vi "AB_API Can Add.vi"(7 "top tree? (true)":bool=TRUE, 8 "error in (no error)":errorcluster, 10 "AB_Source in":refnum<class "AB_Source.lvclass">, 11 "Build in":refnum<class "AB_Build.lvclass">) -> (0 "error out":errorcluster, 1 "can add?":bool, 2 "AB_Source out":refnum<class "AB_Source.lvclass">, 3 "Build out":refnum<class "AB_Build.lvclass">)   [LabVIEW 2020]
uses:
  <vilib>/AppBuilder/AB_Classes/Source/AB_Source.lvclass
  <vilib>/AppBuilder/AB_Classes/Build/AB_Build.lvclass
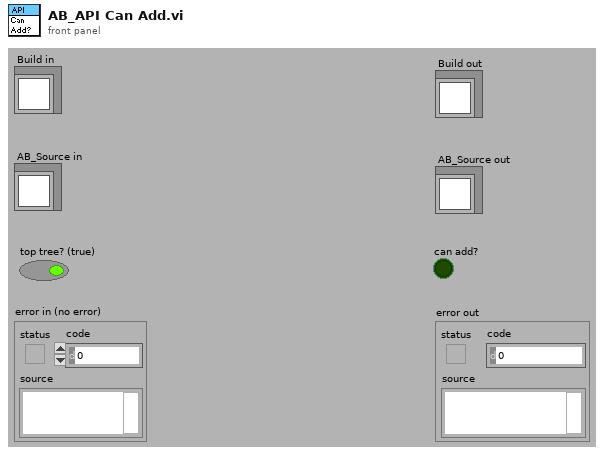
[diagram p1: front panel]
types:
  T1 = typedef "AB_Source.ctl" = cluster{"path":path, "itemID":string, "parentIndex":i32, "sourceInclusion":T2, "destinationIndex":i32, "properties":T3[], "newName":string, "lvfile":bool, "valid":bool, "eng_inBuild":bool, "eng_isNonVILink":bool, "Amalgamation":bool, "Amalgamation Piece":bool, "eng_delimitedName":string, "preventRename":bool}
  T2 = typedef "AB_Source_Inclusion.ctl" = enum16{"IncludeIfReferenced", "Include", "Exclude", "TopLevel"}
  T3 = typedef "AB_Source_Properties.ctl" = cluster{"sourcePropertyType":T4, "value":variant}
  T4 = typedef "AB_Source_Property_Type.ctl" = enum16{"Remove block diagram", "Remove front panel", "Password", "Window has title bar", "Show menu bar", "Show vertical scroll bar", "Show horizontal scroll bar", "Show toolbar", "Show Abort button", "Show fp when called", "Window behavior", "Allow user to close window", "Window run-time position", "Run when opened", "Allow debugging", "Auto error handling", "Generate guard code", "Use stack variables", "Expression folding", "Integer only", "Inline subVI"}
  T5 = typedef "AB_Build.ctl" = cluster{"buildSpecName":string, "buildSpecDescription":string, "destinations":refnum<class "AB_Destination.lvclass">[], "exclusionOption":T6, "defaultLanguage":string, "supportedLanguages":string[], "excludedDirectories":path[], "buildContext":refnum<vi>, "buildObject":T7, "preview":bool, "programatic":bool, "progressBarEvents":T8, "userLog_Path":path, "preActionID":string, "preAction_Path":path, "postActionID":string, "postAction_Path":path, "eng_checkForBrokenVIs?":bool, "eng_verboseLinkerErrors?":bool, "localDest_Path":path, "targetDest_Path":path, "removeVIObject":u16, "cache":refnum<class "PreviewCache.lvclass">, "use cache":bool, "previewCache_ID":string, "buildCache_ID":string, "eng_TempLocalDest_Path":path, "eng_collectDependencies?":bool, "versionInfo":cluster{"buildVersion":cluster{"major":u16, "minor":u16, "patch":u16, "build":u16}, "autoIncrement":bool}, "eng_enableVIChecksums":bool}
  T6 = typedef "AB_Exclusion_Option.ctl" = cluster{"typedefs":bool, "polymorphicVIs":bool, "unusedLibraryItems":bool, "modifyLibraryFile":bool, "edit-timeDependencies":bool, "inlineVIs":bool, "dependent PPLs":bool, "dependent DLLs":bool}
  T7 = typedef "ItemRef.ctl" = u64
  T8 = typedef "provcom_ProgressBar_Events.ctl" = cluster{"newJob":refnum<user-event>, "newItem":refnum<user-event>, "errorMsg":T9, "cancel":refnum<user-event>}
  T9 = typedef "mxLvBuildError.ctl" = refnum<user-event>
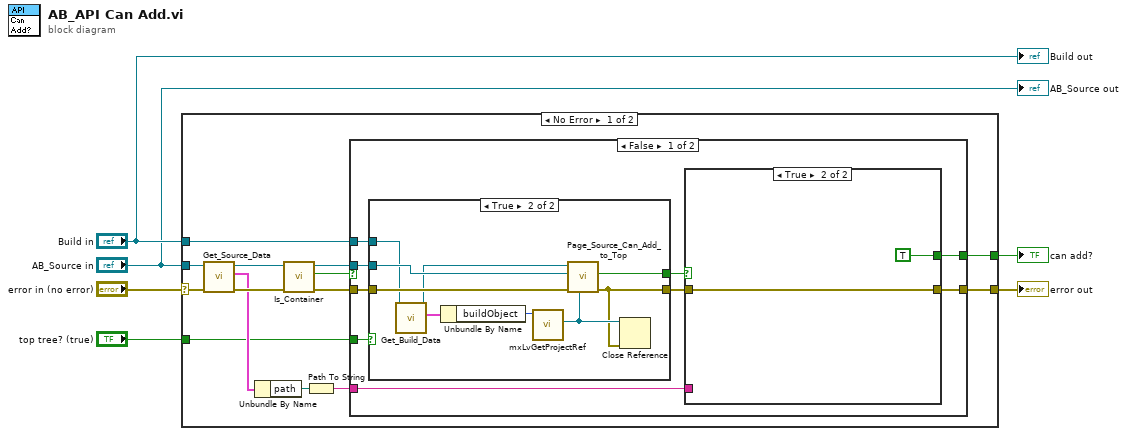
[diagram p0: block diagram]
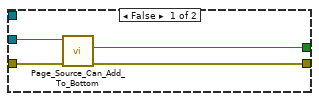
[diagram p2: hidden frame]
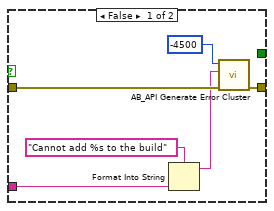
[diagram p3: hidden frame]
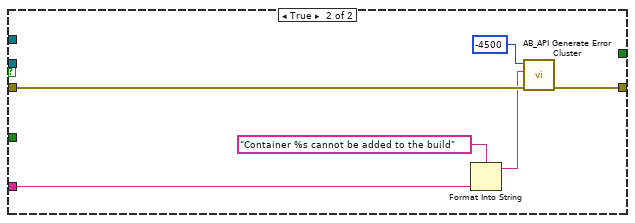
[diagram p4: hidden frame]
diagram:
  n1 = case shown="No Error" "error in (no error)" {
    selector: "error in (no error)" -> [w13 w57]
    tunnel: "Build in" -> [w17 _]
    tunnel: "AB_Source in" -> [w16 _]
    tunnel: [w9 w57] -> w5
    tunnel: [w8 _] -> w4
    tunnel: "top tree? (true)" -> [w7 _]
    frame No Error {
      n2 = call <vilib>:"Get_Source_Data.vi"("error in (no error)"=w13, "Class in"=w16) -> ("error out"=w14:errorcluster, "data"=w12:T1, "Class out"=w15:refnum<class "AB_Source.lvclass">)  [unwired: 7 in]
      n3 = Unbundle By Name(w12) -> ("path"=w11:path)
      n4 = call-dynamic "Is_Container.vi"("error in (no error)"=w14, "AB_Source in"=w15) -> ("error out"=w19:errorcluster, "container"=w20:bool, "AB_Source out"=w18:refnum<class "AB_Source.lvclass">)  [unwired: 7 in]
      n5 = Path To String(path=w11) -> (string=w10:string)
      n6 = case shown="False" w20 {
        tunnel: w19 -> [w26 w55]
        tunnel: [w29 w54] -> w9
        tunnel: w18 -> [w24 _]
        tunnel: w17 -> [w25 _]
        tunnel: w10 -> [w28 w52]
        tunnel: [w27 _] -> w8
        tunnel: w7 -> [w21 _]
        frame False {
          n7 = case shown="True" w21 {
            tunnel: w25 -> [_ w37]
            tunnel: w26 -> [w30 w42]
            tunnel: [w31 w34] -> w23
            tunnel: w24 -> [w33 w40]
            tunnel: [w32 w41] -> w22
            frame False {
              n8 = call-dynamic "Page_Source_Can_Add_To_Bottom.vi"("error in (no error)"=w30, "AB_Source in"=w33) -> ("error out"=w31:errorcluster, "canAddToBottom"=w32:bool)  [unwired: 6 in, 2 out]
            }
            frame True {
              n9 = call <vilib>:"Get_Build_Data.vi"("Class in"=w37) -> ("data"=w38:T5, "Class out"=w36:refnum<class "AB_Build.lvclass">)  [unwired: 1 in, 8 out]
              n10 = Unbundle By Name(w38) -> ("buildObject"=w39:T7)
              n11 = call <resource>:"mxLvGetProjectRef.vi"("Item"=w39) -> ("Project Refnum"=w35:refnum<vi>)  [unwired: 1 in, 9 out]
              n12 = call-dynamic "Page_Source_Can_Add_to_Top.vi"("Project Refnum"=w35, "error in (no error)"=w42, "AB_Source in"=w40, "AB_Build in"=w36) -> ("error out"=w34:errorcluster, "canAddToTop"=w41:bool)  [unwired: 4 in, 2 out]
              n13 = Close Reference(reference=w35, error in (no error)=w34) -> ()  [unwired: 1 out]
            }
          }
          n14 = case shown="True" w22 {
            tunnel: w23 -> [w48 w50]
            tunnel: [w47 w50] -> w29
            tunnel: w28 -> [w43 _]
            tunnel: [_ TRUE] -> w27
            frame False {
              n15 = Format Into String(format string="Cannot add %s to the build", w43) -> (resulting string=w44:string)  [unwired: 2 in, 1 out]
              n16 = call <vilib>:"AB_API Generate Error Cluster.vi"("error in (no error)"=w48, "Additional Message"=w44, "Code"=-4500) -> ("error out"=w47:errorcluster)  [unwired: 8 in]
            }
            frame True {
            }
          }
        }
        frame True {
          n17 = Format Into String(format string="Container %s cannot be added to the build", w52) -> (resulting string=w51:string)  [unwired: 2 in, 1 out]
          n18 = call <vilib>:"AB_API Generate Error Cluster.vi"("error in (no error)"=w55, "Additional Message"=w51, "Code"=-4500) -> ("error out"=w54:errorcluster)  [unwired: 8 in]
        }
      }
    }
    frame Error {
    }
  }
  "error out" <- w5
  "can add?" <- w4
  "Build out" <- "Build in"
  "AB_Source out" <- "AB_Source in"
